vi "Sequence Dialog.vi"(8 "error in (no error)":errorcluster, 10 "Sequence UI":refnum<queue>, 11 "State Cluster In":T3 {"Main Config"."PR Module Configs"."Settings"."PID 2 Parameters"."output range"."output low" format="%.2f"; "Main Config"."PR Module Configs"."Settings"."PID 2 Parameters"."output range"."output high" min=0.0 max=100.0 format="%.2f"; "Main Config"."PR Module Configs"."Settings"."PID 2 Parameters"."PID gains"."derivative time (Td, min)" format="%.3f"; "Main Config"."PR Module Configs"."Settings"."PID 2 Parameters"."PID gains"."integral time (Ti, min)" format="%.3f"; "Main Config"."PR Module Configs"."Settings"."PID 2 Parameters"."PID gains"."proportional gain (Kc)" format="%.3f"; "Main Config"."Steps"."Control" items=["Pump %", "Setpoint"]; "Main Config"."TCU Module Configs"."Settings"."Julabo FP-50 Settings"."Pump Power" min=0 max=8 step=1; "Main Config"."TCU Module Configs"."Settings"."Lauda Settings"."Pump Power" min=0 max=8 step=1; "Main Config"."Pump Module Configs"."Settings"."ASIA Pump C"."channel" min=0 max=1 step=1; "Main Config"."Pump Module Configs"."Settings"."Masterflex"."Pump Number" min=1.0 max=20.0 step=1.0; "Main Config"."Pump Module Configs"."Settings"."Ismatech"."Pump Number" min=1.0 max=20.0 step=1.0; "Main Config"."Feed Module Configs"."Settings"."output range"."output low" min=0.0 max=100.0 format="%.2f"; "Main Config"."Feed Module Configs"."Settings"."output range"."output high" format="%.2f"; "Main Config"."Feed Module Configs"."Settings"."PID 2 Parameters"."PID gains"."derivative time (Td, min)" format="%.3f"; "Main Config"."Feed Module Configs"."Settings"."PID 2 Parameters"."PID gains"."integral time (Ti, min)" format="%.3f"; "Main Config"."Feed Module Configs"."Settings"."PID 2 Parameters"."PID gains"."proportional gain (Kc)" format="%.3f"; "Main Config"."Feed Module Configs"."Settings"."ASIA Pump C"."channel" min=0 max=1 step=1; "Main Config"."Feed Module Configs"."Settings"."Ismatech"."Pump Number" min=1.0 max=20.0 step=1.0; "Main Config"."Feed Module Configs"."Settings"."Masterflex"."Pump Number" min=1.0 max=20.0 step=1.0}) -> (0 "error out":errorcluster, 1 "Start":bool, 2 "cancelled":bool, 3 "State Cluster Out":T3 {"Main Config"."PR Module Configs"."Settings"."PID 2 Parameters"."output range"."output low" format="%.2f"; "Main Config"."PR Module Configs"."Settings"."PID 2 Parameters"."output range"."output high" min=0.0 max=100.0 format="%.2f"; "Main Config"."PR Module Configs"."Settings"."PID 2 Parameters"."PID gains"."derivative time (Td, min)" format="%.3f"; "Main Config"."PR Module Configs"."Settings"."PID 2 Parameters"."PID gains"."integral time (Ti, min)" format="%.3f"; "Main Config"."PR Module Configs"."Settings"."PID 2 Parameters"."PID gains"."proportional gain (Kc)" format="%.3f"; "Main Config"."Steps"."Control" items=["Pump %", "Setpoint"]; "Main Config"."TCU Module Configs"."Settings"."Julabo FP-50 Settings"."Pump Power" min=0 max=8 step=1; "Main Config"."TCU Module Configs"."Settings"."Lauda Settings"."Pump Power" min=0 max=8 step=1; "Main Config"."Pump Module Configs"."Settings"."ASIA Pump C"."channel" min=0 max=1 step=1; "Main Config"."Pump Module Configs"."Settings"."Masterflex"."Pump Number" min=1.0 max=20.0 step=1.0; "Main Config"."Pump Module Configs"."Settings"."Ismatech"."Pump Number" min=1.0 max=20.0 step=1.0; "Main Config"."Feed Module Configs"."Settings"."output range"."output low" min=0.0 max=100.0 format="%.2f"; "Main Config"."Feed Module Configs"."Settings"."output range"."output high" format="%.2f"; "Main Config"."Feed Module Configs"."Settings"."PID 2 Parameters"."PID gains"."derivative time (Td, min)" format="%.3f"; "Main Config"."Feed Module Configs"."Settings"."PID 2 Parameters"."PID gains"."integral time (Ti, min)" format="%.3f"; "Main Config"."Feed Module Configs"."Settings"."PID 2 Parameters"."PID gains"."proportional gain (Kc)" format="%.3f"; "Main Config"."Feed Module Configs"."Settings"."ASIA Pump C"."channel" min=0 max=1 step=1; "Main Config"."Feed Module Configs"."Settings"."Ismatech"."Pump Number" min=1.0 max=20.0 step=1.0; "Main Config"."Feed Module Configs"."Settings"."Masterflex"."Pump Number" min=1.0 max=20.0 step=1.0}, 4 "Pause":bool, 5 "Abort":bool)   [LabVIEW 2018, in "Sequencing Library.lvlib"]
uses:
  Sequencing Library.lvlib
  Squence Control.ctl
  controls/Step Cluster.ctl
  Drag and Drop/State Cluster.ctl
  support/Message Queue/Message Cluster.ctl
  Drag and Drop/Thumbnail Cluster.ctl
  Drag and Drop/Object Cluster.ctl
  <vilib>/Utility/miscctls.llb/LVRectTypeDef.ctl
  Drag and Drop/Object Type Enum.ctl
  <vilib>/Utility/miscctls.llb/LVPositionTypeDef.ctl
  Config Module/Controls/Main Config Cluster.ctl
  OPC/OPC Module Config.ctl
  Scale Module Folder/Measure Instrument/State Enum.ctl
  <vilib>/Utility/miscctls.llb/LVPoint32TypeDef.ctl
  OPC/OPC Settings.ctl
  OPC/Variable Data Cluster.ctl
  <vilib>/OPCUA/controls/NodeId.ctl
  <vilib>/OPCUA/controls/OPC UA StatusCode.ctl
  <vilib>/OPCUA/controls/Subscription ID.ctl
  <vilib>/OPCUA/controls/OPC UA Client Refnum.ctl
  <vilib>/OPCUA/controls/Subscription Data Change.ctl
  <vilib>/OPCUA/controls/Data Type.ctl
  Feed Module/Controls/Feed Module Config Cluster.ctl
  Feed Module/Controls/Feed Module Settings Cluster.ctl
  Ismatec ISM 831C/Controls/Ismatech Settings Cluster.ctl
  Masterflex 7550-30/Controls/Settings Cluster.ctl
  Mettler Toledo/Controls/Settings Cluster.ctl
  Bronkhorst M13 Flow Meter/Settings Cluster.ctl
  Measure Instrument/PID 2 Parameters Cluster.ctl
  Measure Instrument/PID Input Enum.ctl
  Measure Instrument/PID 2 Output Enum.ctl
  Tacmina QI/Tacmina QI DAQ Setting.ctl
  KNF Pump/Settings Cluster plus SIMDOS.ctl
  ASIA Pump/Pump Settings.ctl
  VICI M50 Party Mode/Settings Cluster.ctl
  FLOM Pump/Settings Cluster.ctl
  SSI PR Class/SSI PR or LD Settings Cluster.ctl
  Masterflex 75211/Masterflex 75211 DAQ Setting.ctl
  SSI PR Class/SSI P40 Settings Cluster.ctl
  TT Module/Controls/TT Module Config Cluster.ctl
  Tag VIs/Numeric Alarm Settings Cluster.ctl
  Acquisition/Hardware Configuration.ctl
  Acquisition/Task Cluster.ctl
  PT Module/Controls/PT Module Config Cluster.ctl
  Scale Module Folder/Feed Module/Controls/Scale Module Config Cluster.ctl
  Scale Module Folder/Feed Module/Controls/Scale Module Settings Cluster.ctl
  Pump Module Folder/Pump Module Config Cluster.ctl
  Pump Module Folder/Pump Module Settings Cluster.ctl
  LabJack Module/Controls/U3 Module Config Cluster.ctl
  Decoration Module/Decoration Module Config Cluster.ctl
  Flow Module Folder/Feed Module/Controls/Flow Module Config Cluster.ctl
  Flow Module Folder/Feed Module/Controls/Flow Module Settings Cluster.ctl
  TCU Module/TCU Module Folder/TCU Module Config Cluster.ctl
  TCU Module/TCU Module Folder/TCU Module Settings Cluster.ctl
  TCU Module/TCU Module Folder/Measure Instrument/Output Devices.ctl
  Huber TCU/Huber Settings.ctl
  Lauda Integral XT-150 TCU/Lauda Settings.ctl
  Julabo Type 1 TCU/Julabo Type 1 TCU Folder/Julabo FP-50 Settings.ctl
  Huber Unistat 410 TCU/Huber Unistat 410 Settings.ctl
  D-O Module Folder/Not Sure Where this is Used.ctl
  D-O Module Folder/D-O Module Config Cluster.ctl
  D-O Module Folder/Valve Clusters.ctl
  D-O Module Folder/D-O Module Settings Cluster.ctl
  D-O Module Folder/D-O Device Settings Cluster.ctl
  VICI Electronic Actuator/VICI Electronic Actuator Settings.ctl
  Pressure Regulator Control Module/Pressure Regulator/Controls/4-20mA Module Config Cluster.ctl
  Pressure Regulator Control Module/Pressure Regulator/Controls/4-20mA Module Settings Cluster.ctl
  Pressure Transmitter/Pressure Transmitter Device Settings.ctl
  Pressure Reg Module/Pressure Regulator Device Settings.ctl
  support/Message Queue/Enqueue Message (Single).vi
  support/Message Queue/Message Queue.lvlib
  Drag and Drop/Drag and Drop.lvlib
  Config Module/Config Module.lvlib
  TT Module/TT Module.lvlib
  Feed Module/Feed Module.lvlib
  Ismatec ISM 831C/Ismatec ISM 831C.lvlib
  Masterflex 7550-30/Masterflex 7550-30.lvlib
  Mettler Toledo/Mettler Toledo.lvlib
  Bronkhorst M13 Flow Meter/Bronkhorst M13 Flow Meter.lvlib
  Tacmina QI/Tacmina QI.lvlib
  KNF Pump/KNF SIMDOS.lvlib
  ASIA Pump.lvlib
  DAQ/DAQ.lvlib
  PT Module/PT Module.lvlib
  Scale Module Folder/Scale Module.lvlib
  Pump Module Folder/Pump Module.lvlib
  LabJack Module/U3 Module.lvlib
  Flow Module Folder/Flow Module.lvlib
  TCU Module/TCU Module Folder/TCU Module.lvlib
  Huber TCU/Huber Ministat 230 TCU.lvlib
  Lauda Integral XT-150 TCU/Lauda TCU.lvlib
  Julabo Type 1 TCU/Julabo Type 1 TCU Folder/Julabo Type FP-50 TCU.lvlib
  VICI M50 Party Mode/VICI M6 M50 Party Mode.lvlib
  D-O Module Folder/D-O Module.lvlib
  Pressure Transmitter/Pressure Transmitter Library.lvlib
  Pressure Regulator Control Module/Pressure Regulator/4-20mA Module.lvlib
  Pressure Reg Module/Pressure Regulator Library.lvlib
  FLOM Pump/FLOM Pump.lvlib
  SSI PR Class/SSI PR or LD Pump.lvlib
  Huber Unistat 410 TCU/Huber Unistat 410 TCU.lvlib
  OPC/OPC UA.lvlib
  Scale Module Folder/Measure Instrument/Scale Module Engine.lvlib
  D-O Module Folder/DIO Valve/VICI Electronic Actuator.lvlib
  Masterflex 75211/Masterflex 75211.lvlib
  SSI PR Class/SSI P40 Pump.lvlib
panel:
  out "Main Config.Steps":T1 {"Control" items=["Pump %", "Setpoint"]}
  out "Strings []":string[](array[string])
  in  "Abort  Button":bool
  in  "Pause Button":bool
  in  "Save Button":bool
  in  "Step Array":T65[](array[typedef]) {"Value" min=0.0 max=100.0; "Control" items=["Pump Module Setpoint", "Feed Module Setpoint", "Digital On/Off", "Wait Until Output <=", "Wait Until Output >=", "TCU Pump Setpoint", "TCU Temperature Setpoint", "Wait until TCU Temp <=", "Wait until TCU Temp >=", "Default"]; "Module" items=["Default", "Start Loop", "End Loop", "PM1"]}
  out "Steps out":T2[](array[typedef]) {"Control" items=["Setpoint", "Pump %"]}
  in  "Cancel Button":bool
  in  "Start Button":bool
  # "Module"
  # "Control"
  # "Value"
  # "Wait (sec)"
  # "Running"
  # "Instrument Settings"
  # "Instrument Settings"
  # "Output Instruments"
  # "Flow Meter Settings"
  # "Output Instruments"
  # "Scale Settings"
  # "Output Instruments"
  # "Input Instruments"
  # "Instrument Settings"
  # "Instrument Settings"
  # "Output Instruments"
  # "Flow Meter Settings"
  # "Output Instruments"
  # "Scale Settings"
  # "Output Instruments"
  # "Input Instruments"
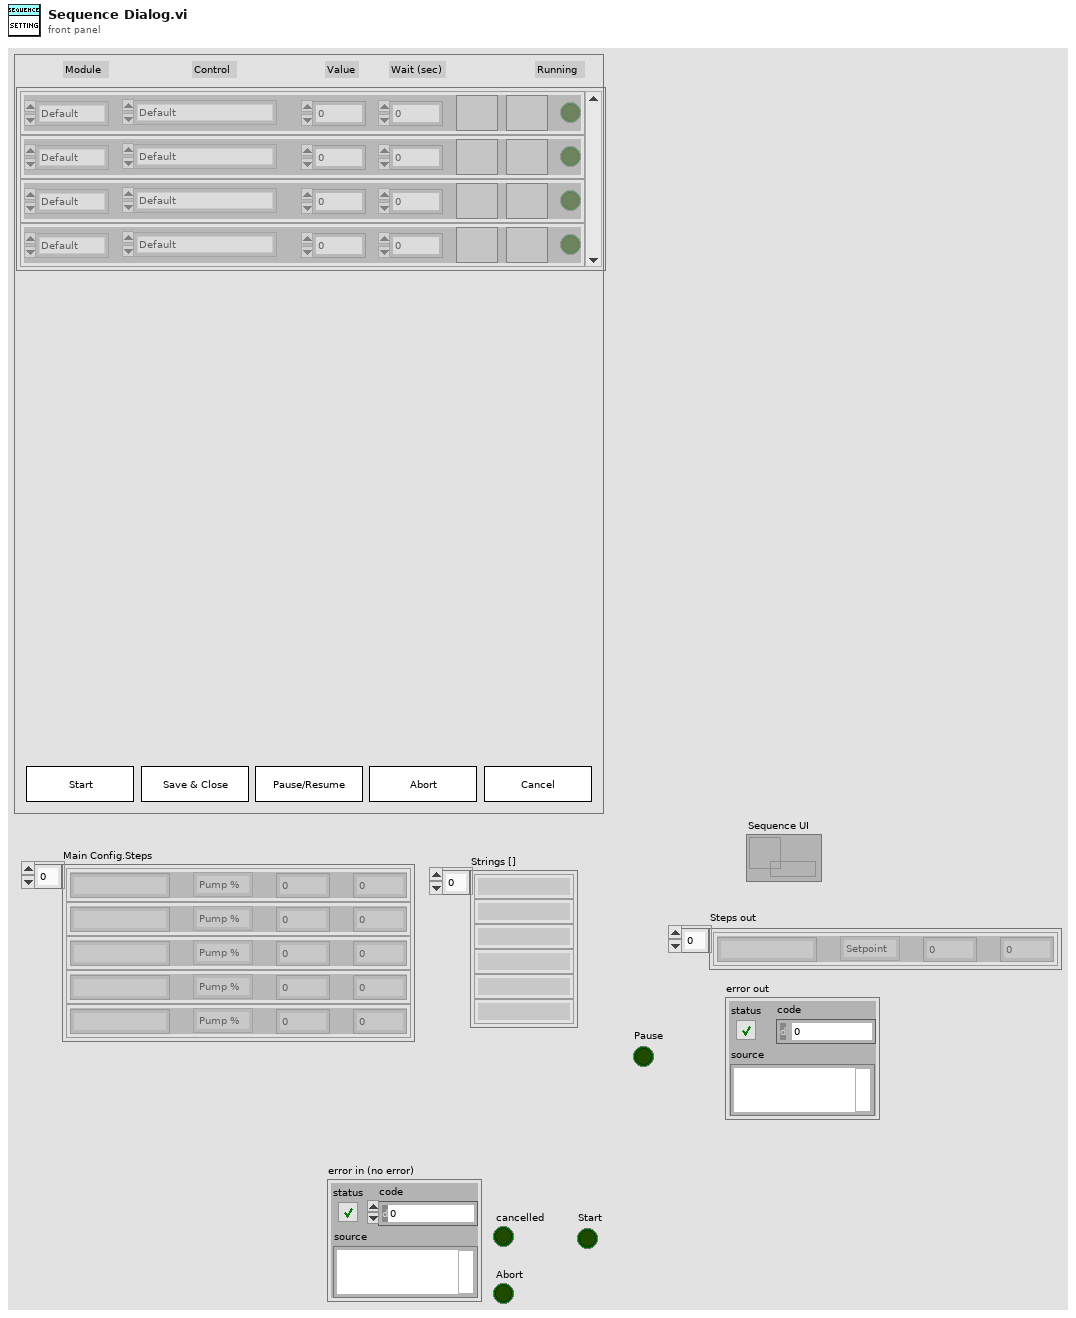
[diagram p1: front panel]
types:
  T1 = typedef "Not Sure Where this is Used.ctl" = T2[]
  T2 = typedef "Sequencing Library.lvlib/Squence Control.ctl" = cluster{"Module":string, "Control":u16, "Value":dbl, "Wait (sec)":dbl}
  T3 = typedef "Drag and Drop.lvlib/State Cluster.ctl" = cluster{"VI refs":refnum<vi>[], "Queues":refnum<queue>[], "[Thumbnails]":T4[], "Drag Object Idx":i32, "[Objects]":T5[], "Active Object":i32, "Drop Offset":T8, "Process Name":string, "Main Config":T9, "Campaign Filepath":path, "Config Changed?":bool}
  T4 = typedef "Thumbnail Cluster.ctl" = cluster{"Path":path, "Rectangle":cluster{"left":i16, "top":i16, "right":i16, "bottom":i16}}
  T5 = typedef "Object Cluster.ctl" = cluster{"BMP Path":path, "Anchor Position":cluster{"X":i32, "Y":i32}, "Hot Spot":T6, "Type":T7, "Parameters":variant}
  T6 = typedef "LVRectTypeDef.ctl" = cluster{"Left":i16, "Top":i16, "Right":i16, "Bottom":i16}
  T7 = typedef "Object Type Enum.ctl" = enum16{"Icon", "Line", "Text", "Feed Module"}
  T8 = typedef "LVPositionTypeDef.ctl" = cluster{"Left":i32, "Top":i32}
  T9 = typedef "Config Module.lvlib/Main Config Cluster.ctl" = cluster{"Notebook":string, "Page":string, "OPC Module Configs":T10[], "Feed Module Configs":T19[], "Log File Path":path, "TT Module Configs":T36[], "DAQ Config":T38, "PT Module Configs":T40[], "Scale Module Configs":T41[], "Pump Module Configs":T43[], "U3 Module Configs":T45[], "Decoration Module Configs":T46[], "Flow Module Configs":T47[], "TCU Module Configs":T49[], "Steps":T1, "Abort":bool, "DO Module Configs":T56[], "PR Module Configs":T61[], "Cycle Period":dbl}
  T10 = typedef "OPC UA.lvlib/OPC Module Config.ctl" = cluster{"State":T11, "GUID":string, "Drop Coords":T12, "Configuration":T13, "First Iteration":bool, "Data":cluster{"Object Name":string, "Variable Array":T14[]}[], "Process Name":string, "Load Count":i32, "Log Started":bool, "subscription ID out":T17, "OPC UA client refnum out":T18, "Event Registration Refnum":refnum<event-registration>, "Start Time":timestamp, "Current Time":timestamp}
  T11 = typedef "Scale Module.lvlib/Scale Module Engine.lvlib/State Enum.ctl" = enum16{"Measuring", "Idle"}
  T12 = typedef "LVPoint32TypeDef.ctl" = cluster{"Horizontal":i32, "Vertical":i32}
  T13 = typedef "OPC UA.lvlib/OPC Settings.ctl" = cluster{"Cycle Period":dbl, "server endpoint URL":string, "security policy":cluster{"message mode":enum16{"None", "Sign", "Sign and Encrypt"}, "security":enum16{"Basic256", "Basic128Rsa15"}}, "Trust Any Server":bool}
  T14 = typedef "OPC UA.lvlib/Variable Data Cluster.ctl" = cluster{"node ID":T15, "browse name":string, "status":T16, "timestamp":timestamp, "value ":variant}
  T15 = typedef "NodeId.ctl" = string
  T16 = typedef "OPC UA StatusCode.ctl" = u32
  T17 = typedef "Subscription ID.ctl" = u32
  T18 = typedef "OPC UA Client Refnum.ctl" = refnum<k21>
  T19 = typedef "Feed Module.lvlib/Feed Module Config Cluster.ctl" = cluster{"GUID":string, "Drop Coords":T12, "Process Name":string, "Queue Name":string, "Settings":T20, "Settings Load Count":i32, "OP Load Count":i32}
  T20 = typedef "Feed Module.lvlib/Feed Module Settings Cluster.ctl" = cluster{"Cycle Period":dbl, "Ismatech":T21, "Masterflex":T22, "Mettler":T23, "Bronkhorst M13 Flow Meter":T24, "PID 2 Parameters":T25, "Manual Entry":dbl, "Auto?":bool, "output range":cluster{"output high":dbl, "output low":dbl}, "Bronkhorst M14":T23, "Tacmina Settings":T28, "KNF SIMDOS Settings":T29, "ASIA Pump C":T30, "VICI Settings":T31, "FLOM Settings":T32, "SSI PR/LD Settings":T33, "Masterflex 75211 Settings":T34, "SSI P40 Settings":T35}
  T21 = typedef "Ismatec ISM 831C.lvlib/Ismatech Settings Cluster.ctl" = cluster{"VISA resource name":refnum<visa-resource-name>, "Simulated?":bool, "Pump Number":dbl, "Reverse?":bool}
  T22 = typedef "Masterflex 7550-30.lvlib/Settings Cluster.ctl" = cluster{"VISA resource name":refnum<visa-resource-name>, "Simulated?":bool, "Pump Number":dbl, "Reverse?":bool}
  T23 = typedef "Mettler Toledo.lvlib/Settings Cluster.ctl" = cluster{"VISA resource name":refnum<visa-resource-name>, "Simulated?":bool}
  T24 = typedef "Bronkhorst M13 Flow Meter.lvlib/Settings Cluster.ctl" = cluster{"VISA resource name":refnum<visa-resource-name>, "Simulated?":bool}
  T25 = typedef "PID 2 Parameters Cluster.ctl" = cluster{"Input Device":T26, "Output Device":T27, "Setpoint":dbl, "PID gains":cluster{"proportional gain (Kc)":dbl, "integral time (Ti, min)":dbl, "derivative time (Td, min)":dbl}}
  T26 = typedef "PID Input Enum.ctl" = enum16{"Default", "Bronkhorst M13", "Bronkhorst M14", "Scale Rate of Change"}
  T27 = typedef "PID 2 Output Enum.ctl" = enum16{"Default", "Ismatec ISM 831C", "Masterflex 7550-30", "VICI", "Tacmina QI", "KNF SIMDOS", "ASIA Type C", "FLOM UI-22-11", "SSI PR/LD", "SSI P40", "Masterflex 75211-70"}
  T28 = typedef "Tacmina QI.lvlib/Tacmina QI DAQ Setting.ctl" = cluster{"Analog DAQ Task":refnum<k21>, "Digital DAQ Task":refnum<k21>}
  T29 = typedef "KNF SIMDOS.lvlib/Settings Cluster plus SIMDOS.ctl" = cluster{"VISA resource name":refnum<visa-resource-name>, "Simulated?":bool}
  T30 = typedef "ASIA Pump.lvlib/Pump Settings.ctl" = cluster{"ASIA Pump #":i32, "channel":i32, "Simulated":bool}
  T31 = typedef "VICI M6 M50 Party Mode.lvlib/Settings Cluster.ctl" = cluster{"VISA resource name":refnum<visa-resource-name>, "Simulated?":bool, "Pump Letter":string, "Reverse?":bool}
  T32 = typedef "FLOM Pump.lvlib/Settings Cluster.ctl" = cluster{"VISA resource name":refnum<visa-resource-name>, "Simulated?":bool, "Pump Number":dbl}
  T33 = typedef "SSI PR or LD Pump.lvlib/SSI PR or LD Settings Cluster.ctl" = cluster{"VISA resource name":refnum<visa-resource-name>, "Simulated?":bool}
  T34 = typedef "Masterflex 75211.lvlib/Masterflex 75211 DAQ Setting.ctl" = cluster{"Analog DAQ Task":refnum<k21>, "Digital DAQ Task":refnum<k21>}
  T35 = typedef "SSI P40 Pump.lvlib/SSI P40 Settings Cluster.ctl" = cluster{"VISA resource name":refnum<visa-resource-name>, "Simulated?":bool}
  T36 = typedef "TT Module.lvlib/TT Module Config Cluster.ctl" = cluster{"GUID":string, "Drop Coords":T12, "Input Channel Tag Name ":string, "Process Name":string, "Queue Name":string, "Input Channel Numeric Alarm Settings":T37[]}
  T37 = typedef "Numeric Alarm Settings Cluster.ctl" = cluster{"enable? (F)":bool, "name":string, "alarm type":enum16{"HI_HI", "HI", "LO", "LO_LO"}, "level/change":dbl, "deadband/time":dbl, "alarm delay":dbl, "priority":u32, "ack type":enum16{"Auto", "User", "None", "Each Occurrence"}, "area":string, "description":string, "log? (T)":bool}
  T38 = typedef "DAQ.lvlib/Hardware Configuration.ctl" = cluster{"Tasks":T39[]}
  T39 = typedef "Task Cluster.ctl" = cluster{"DAQmx Task":refnum<k21>, "Read-Write Radio":enum32{"Read", "Write"}}
  T40 = typedef "PT Module.lvlib/PT Module Config Cluster.ctl" = cluster{"GUID":string, "Drop Coords":T12, "Input Channel Tag Name ":string, "Process Name":string, "Queue Name":string, "Input Channel Numeric Alarm Settings":T37[]}
  T41 = typedef "Scale Module.lvlib/Scale Module Config Cluster.ctl" = cluster{"GUID":string, "Drop Coords":T12, "Process Name":string, "Queue Name":string, "Settings":T42, "Load Count":i32}
  T42 = typedef "Scale Module.lvlib/Scale Module Settings Cluster.ctl" = cluster{"Cycle Period":dbl, "Mettler":T23, "Scale Type":string}
  T43 = typedef "Pump Module.lvlib/Pump Module Config Cluster.ctl" = cluster{"GUID":string, "Drop Coords":T12, "Process Name":string, "Queue Name":string, "Settings":T44, "Load Count":i32}
  T44 = typedef "Pump Module.lvlib/Pump Module Settings Cluster.ctl" = cluster{"Cycle Period":dbl, "Manual Entry":dbl, "Output Device":T27, "Ismatech":T21, "Masterflex":T22, "VICI Settings":T31, "Tacmina Settings":T28, "KNF SIMDOS Settings":T29, "ASIA Pump C":T30, "FLOM Settings":T32, "SSI PR/LD Settings":T33, "SSI P40 Settings":T33, "Masterflex 75211 Settings":T34, "Pump Calibration File":path, "Calibration Slope":dbl, "Calibration Y Intercept":dbl, "Pump Cal Enum":u16}
  T45 = typedef "U3 Module.lvlib/U3 Module Config Cluster.ctl" = cluster{"GUID":string, "Drop Coords":T12, "AI Channel Number":enum16{"Default", "AI0", "AI1", "AI2", "AI3", "AI4", "AI5", "AI6", "AI7"}, "Process Name":string, "Queue Name":string, "Input Channel Numeric Alarm Settings":T37[]}
  T46 = typedef "Decoration Module Config Cluster.ctl" = cluster{"GUID":string, "Drop Coords":T12, "Decoration Filepath":path}
  T47 = typedef "Flow Module.lvlib/Flow Module Config Cluster.ctl" = cluster{"GUID":string, "Drop Coords":T12, "Process Name":string, "Queue Name":string, "Settings":T48, "Load Count":i32}
  T48 = typedef "Flow Module.lvlib/Flow Module Settings Cluster.ctl" = cluster{"Cycle Period":dbl, "Bronkhorst M13":T23, "Flow Meter Type":string, "Bronkhorst M14":T23}
  T49 = typedef "TCU Module.lvlib/TCU Module Config Cluster.ctl" = cluster{"GUID":string, "Drop Coords":T12, "Process Name":string, "Queue Name":string, "Settings":T50, "Load Count":i32, "Power Level Changed":bool}
  T50 = typedef "TCU Module.lvlib/TCU Module Settings Cluster.ctl" = cluster{"Cycle Period":dbl, "Setpoint Entry":dbl, "Output Device":T51, "Huber Ministat 230 Settings":T52, "Lauda Settings":T53, "Julabo FP-50 Settings":T54, "Internal Control?":bool, "Huber Unistat 410 Settings":T55}
  T51 = typedef "Output Devices.ctl" = enum16{"Default", "Huber Ministat 230", "Huber Unistat 410", "Lauda XT-150", "Julabo FP-50"}
  T52 = typedef "Huber Ministat 230 TCU.lvlib/Huber Settings.ctl" = cluster{"VISA resource name":refnum<visa-resource-name>, "Simulated?":bool}
  T53 = typedef "Lauda TCU.lvlib/Lauda Settings.ctl" = cluster{"VISA resource name":refnum<visa-resource-name>, "Simulated?":bool, "Pump Power":i32}
  T54 = typedef "Julabo Type FP-50 TCU.lvlib/Julabo FP-50 Settings.ctl" = cluster{"VISA resource name":refnum<visa-resource-name>, "Simulated?":bool, "Pump Power":i32}
  T55 = typedef "Huber Unistat 410 TCU.lvlib/Huber Unistat 410 Settings.ctl" = cluster{"VISA resource name":refnum<visa-resource-name>, "Simulated?":bool}
  T56 = typedef "D-O Module.lvlib/D-O Module Config Cluster.ctl" = cluster{"GUID":string, "Drop Coords":T12, "Process Name":string, "Queue Name":string, "Settings":T57, "Load Count":i32}
  T57 = typedef "D-O Module.lvlib/Valve Clusters.ctl" = cluster{"Valve Settings":T58, "Valve Type":enum16{"Default", "Digital Output Valve", "VICI Electronic Actuator"}, "Time On (Sec)":dbl, "Time Off (Sec)":dbl, "Run?":bool}
  T58 = typedef "D-O Module.lvlib/D-O Module Settings Cluster.ctl" = cluster{"D-O Settings":T59, "VICI Electronic Actuator":T60}
  T59 = typedef "D-O Module.lvlib/D-O Device Settings Cluster.ctl" = cluster{"DAQmx Task Name":refnum<k21>, "Output Channel":u16, "Output Channel Names":string[]}
  T60 = typedef "VICI Electronic Actuator.lvlib/VICI Electronic Actuator Settings.ctl" = cluster{"VISA resource name":refnum<visa-resource-name>, "Mode":enum16{"Two Positions With Stops", "Two Positions Without Stops", "Mutiposition"}, "Simulated":bool}
  T61 = typedef "4-20mA Module.lvlib/4-20mA Module Config Cluster.ctl" = cluster{"GUID":string, "Drop Coords":T12, "Process Name":string, "Queue Name":string, "Settings":T62, "Settings Load Count":i32}
  T62 = typedef "4-20mA Module.lvlib/4-20mA Module Settings Cluster.ctl" = cluster{"Cycle Period":dbl, "PID 2 Parameters":cluster{"Input Device":enum16{"Default", "4-20mA"}, "Output Device":enum16{"Default", "Equilibar Pressure Reg", "Flow Regulator"}, "Setpoint":dbl, "PID gains":cluster{"proportional gain (Kc)":dbl, "integral time (Ti, min)":dbl, "derivative time (Td, min)":dbl}, "output range":cluster{"output low":dbl, "output high":dbl}}, "Manual Entry":dbl, "Auto?":bool, "4-20mA Input Settings":T63, "4-20mA Out Settings":T64, "Input Channel Tag Name ":string}
  T63 = typedef "Pressure Transmitter Library.lvlib/Pressure Transmitter Device Settings.ctl" = cluster{"Input Channel ":u16}
  T64 = typedef "Pressure Regulator Library.lvlib/Pressure Regulator Device Settings.ctl" = cluster{"Output DAQ Task":refnum<k21>}
  T65 = typedef "Sequencing Library.lvlib/Step Cluster.ctl" = cluster{"Add Button":bool, "Remove Button":bool, "Module":u16, "Control":u16, "Value":dbl, "Wait (sec)":dbl, "Step Running":bool}
  T66 = cluster{"Add Button":bool, "Remove Button":bool, "Module":u16, "Control":u16, "Value":dbl, "Wait (sec)":dbl, "Step Running":bool}
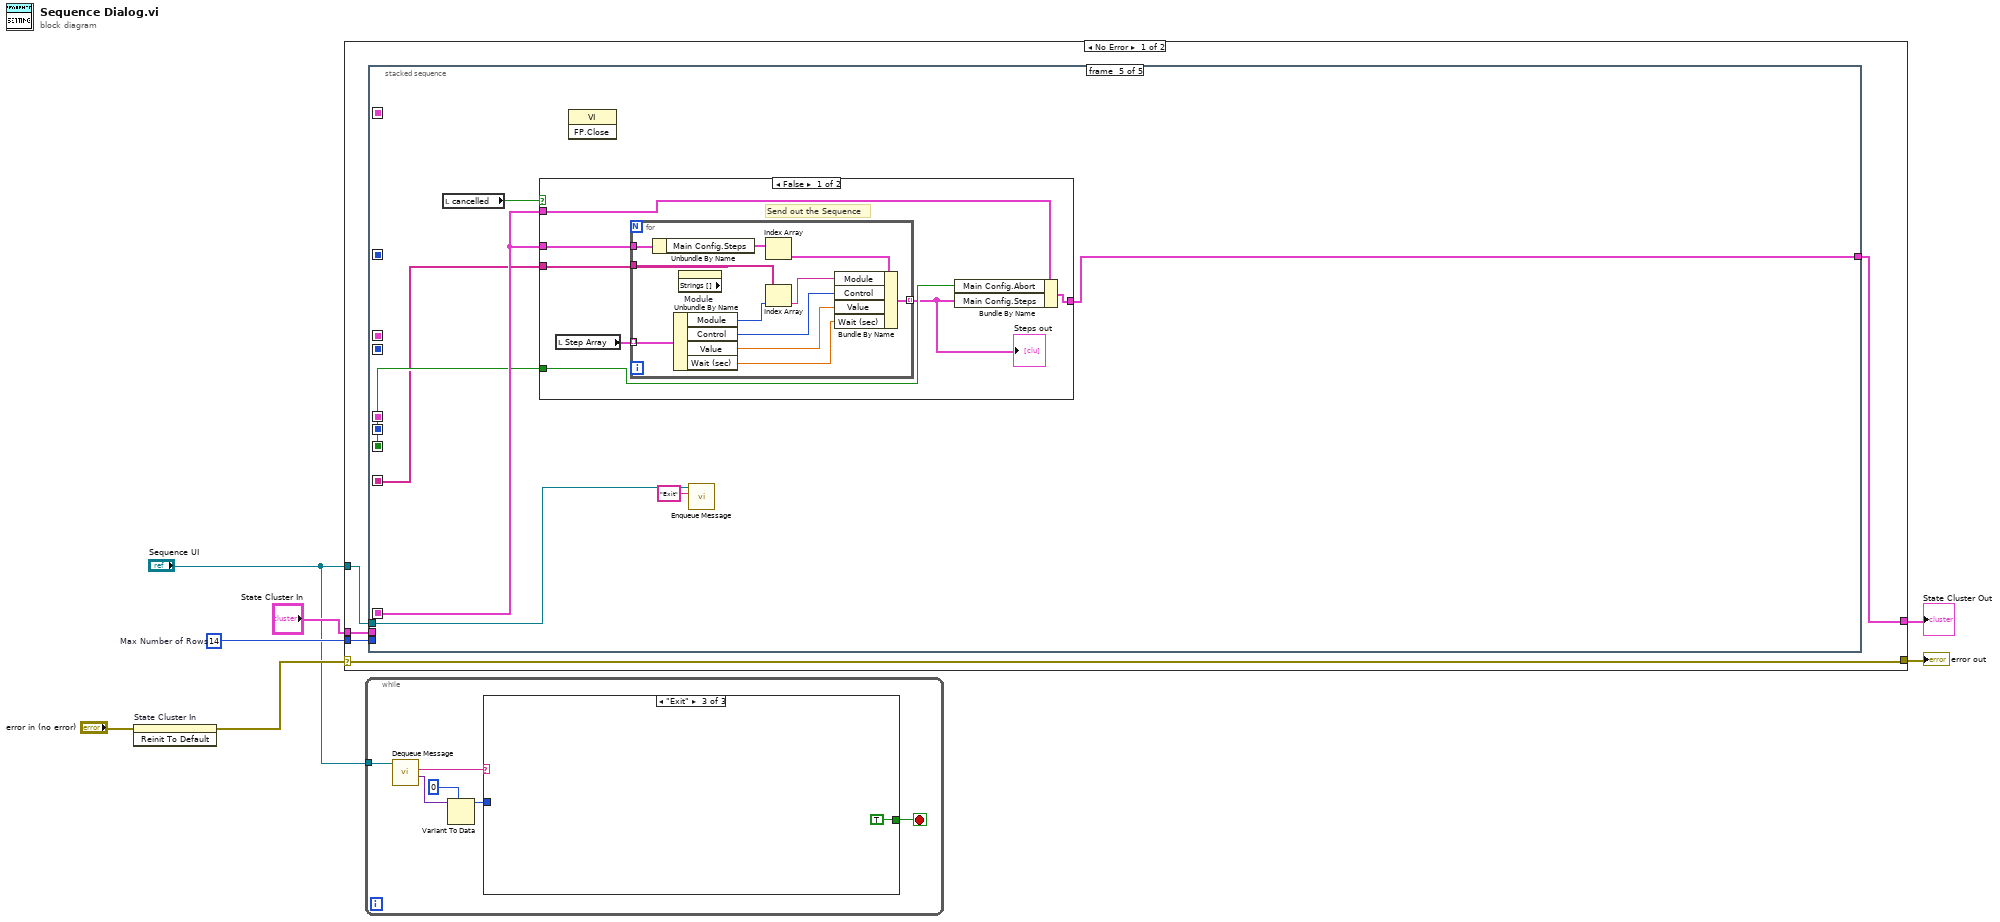
[diagram p0: block diagram]
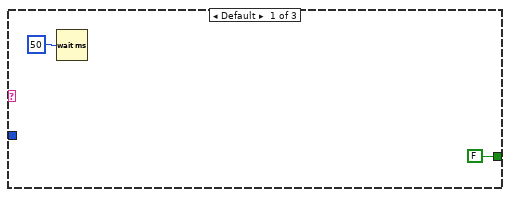
[diagram p2: hidden frame]
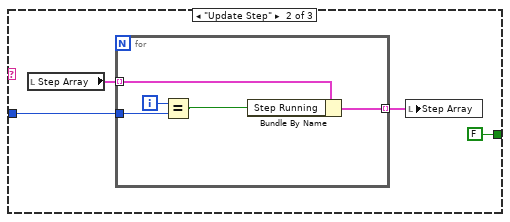
[diagram p3: hidden frame]
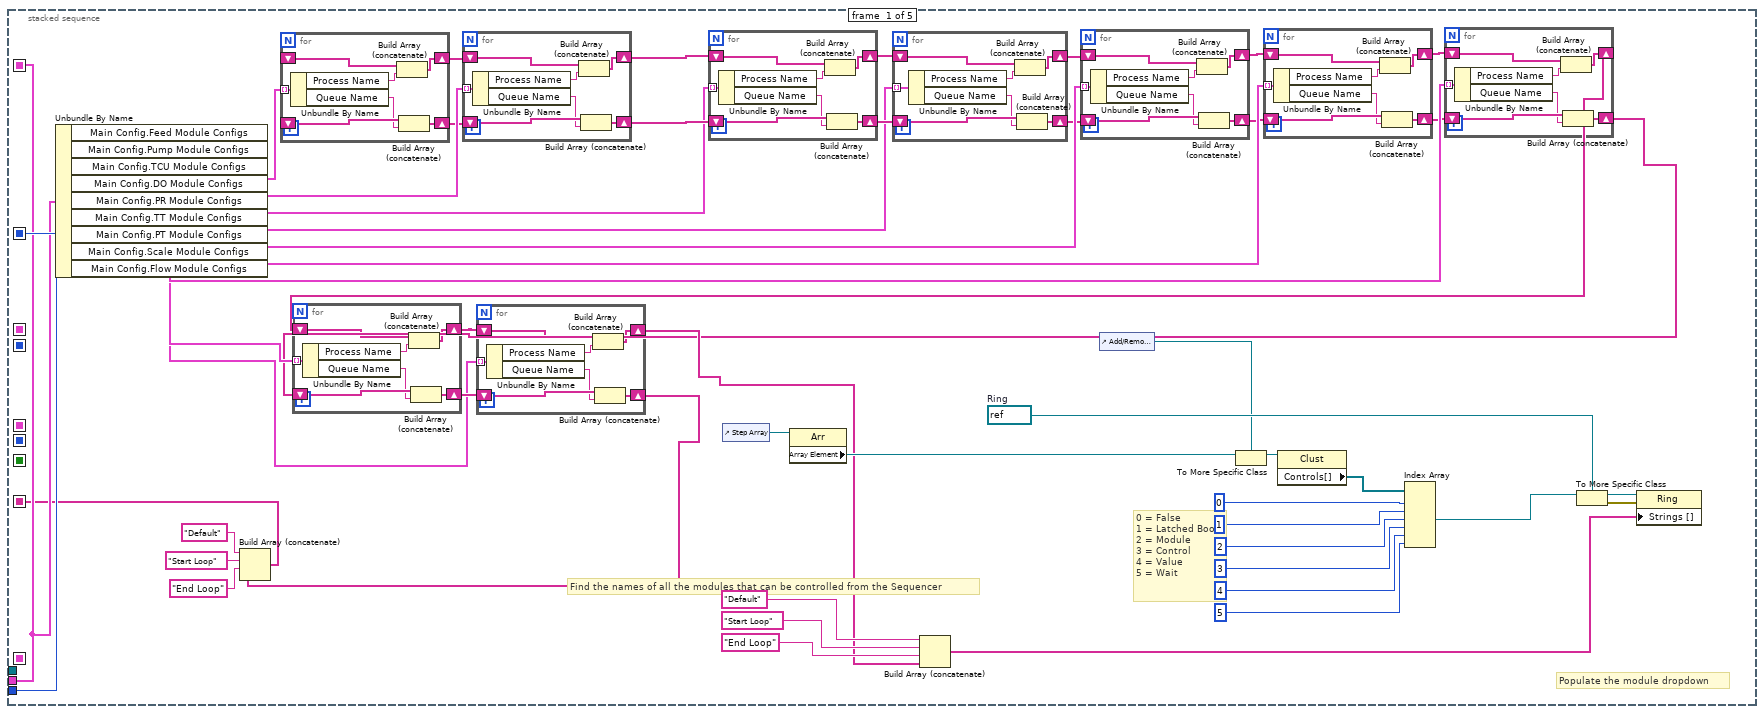
[diagram p4: hidden frame]
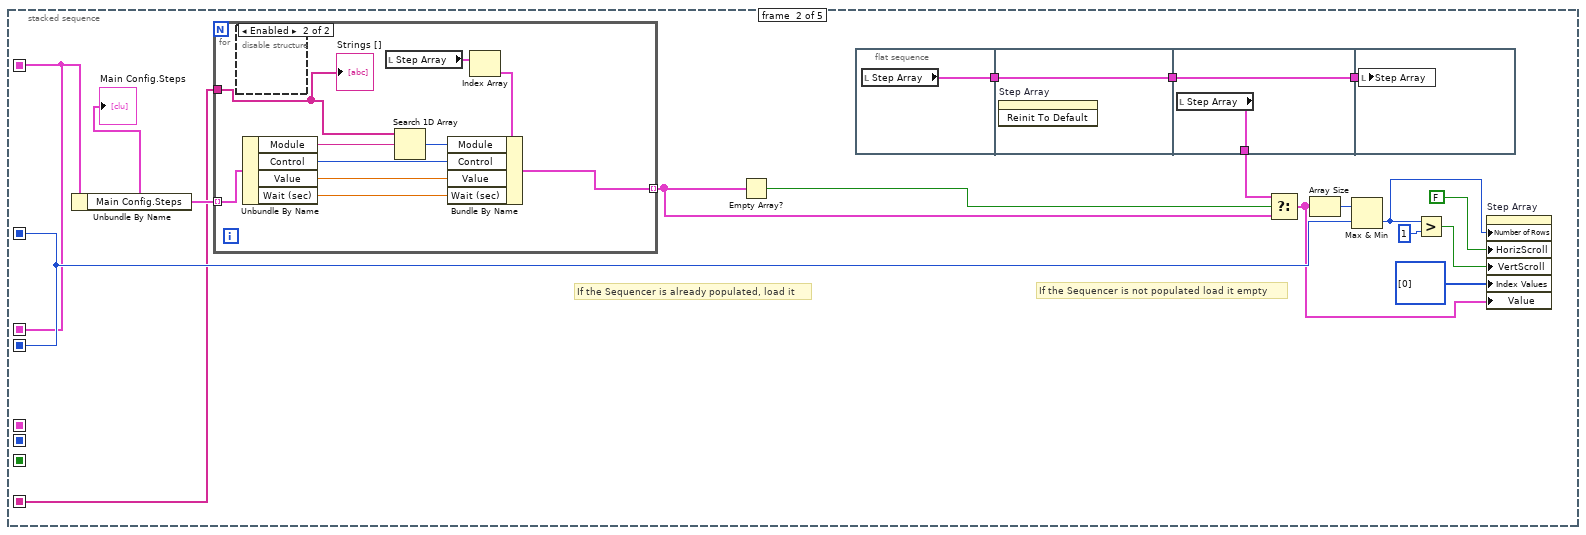
[diagram p5: hidden frame]
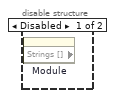
[diagram p6: hidden frame]
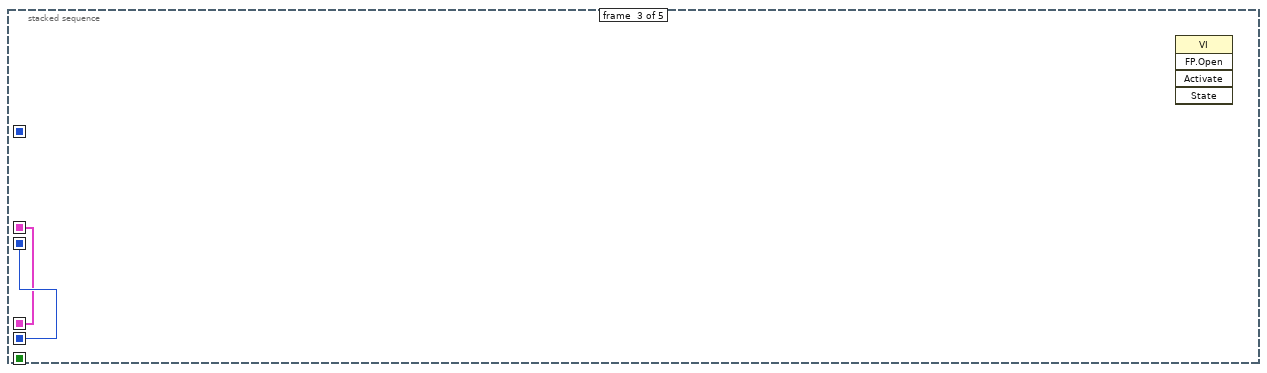
[diagram p7: hidden frame]
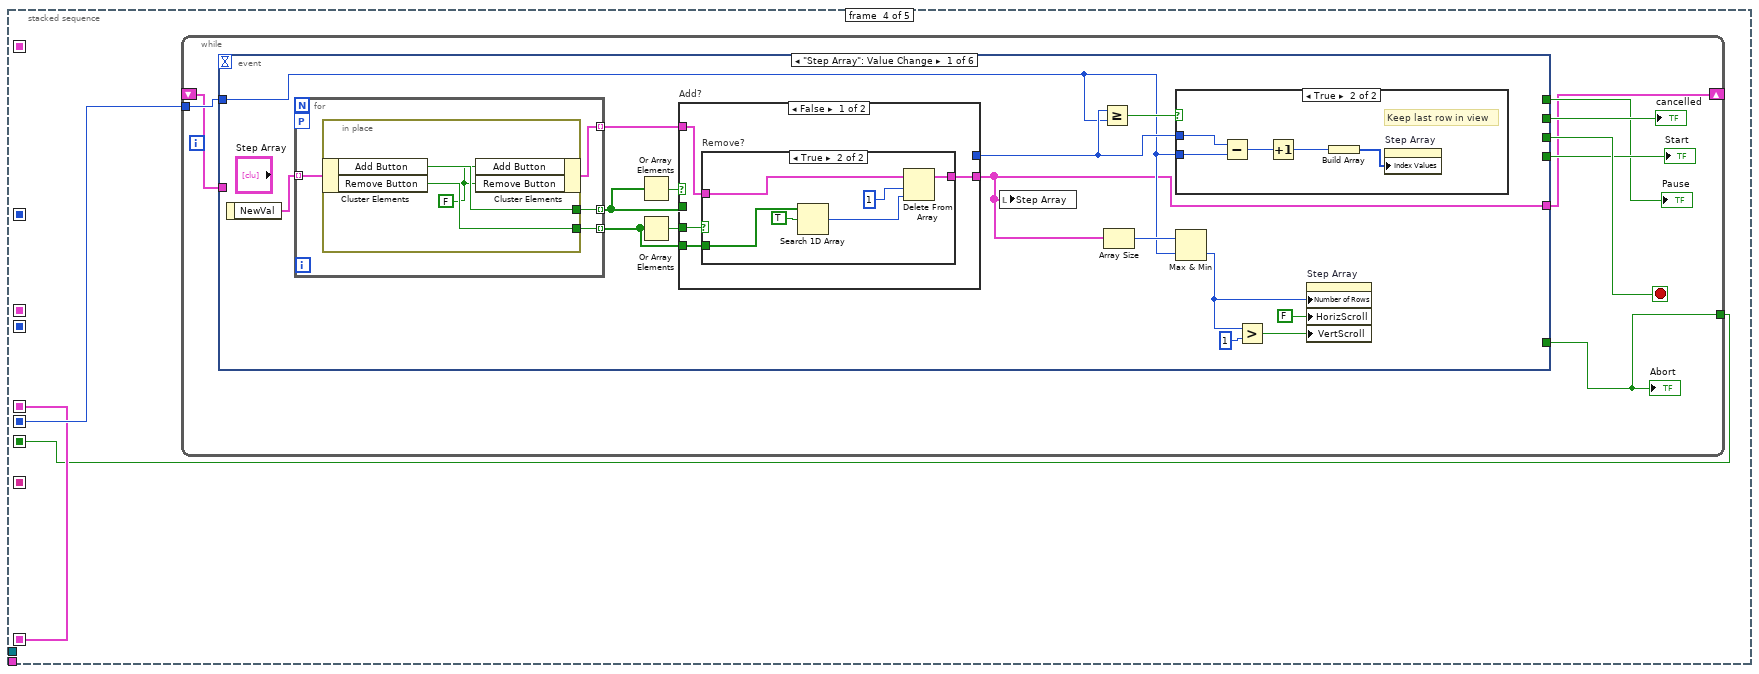
[diagram p8: hidden frame]
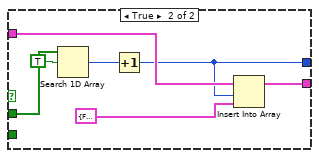
[diagram p11: hidden frame]
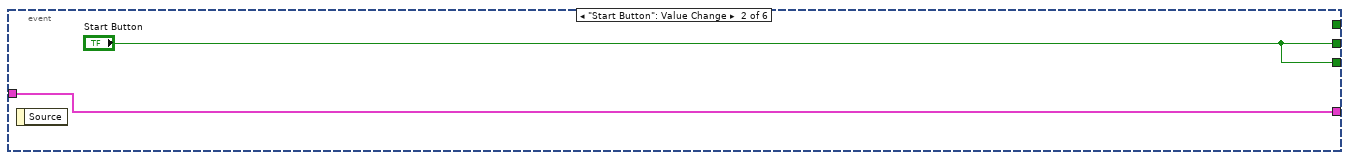
[diagram p12: hidden frame]
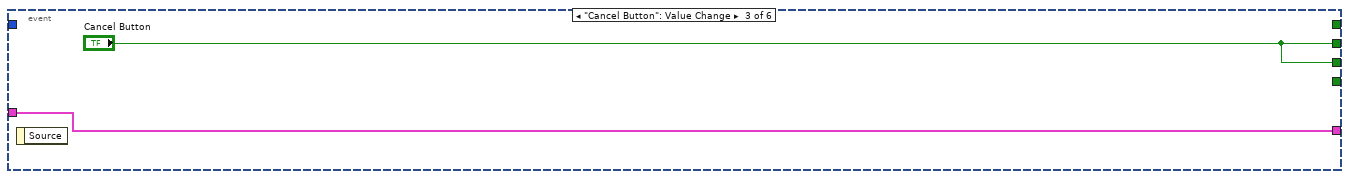
[diagram p13: hidden frame]
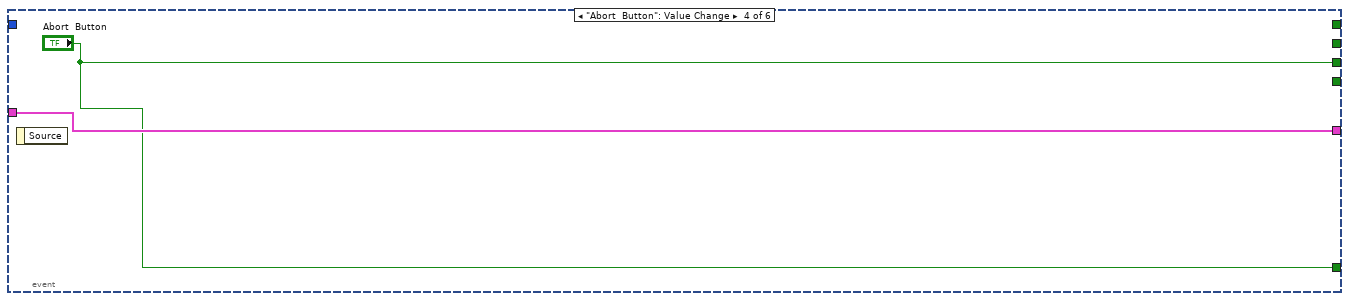
[diagram p14: hidden frame]
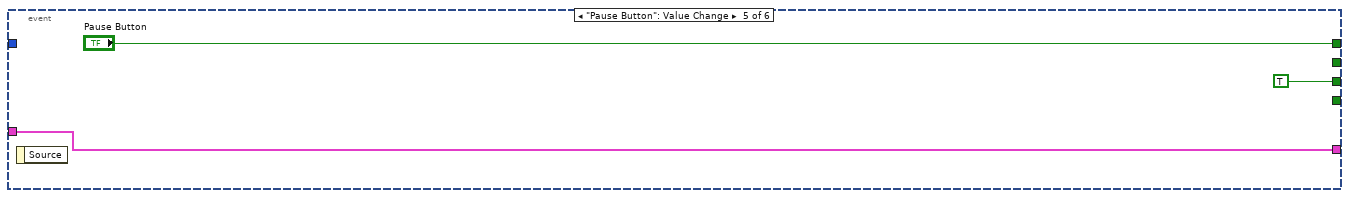
[diagram p15: hidden frame]
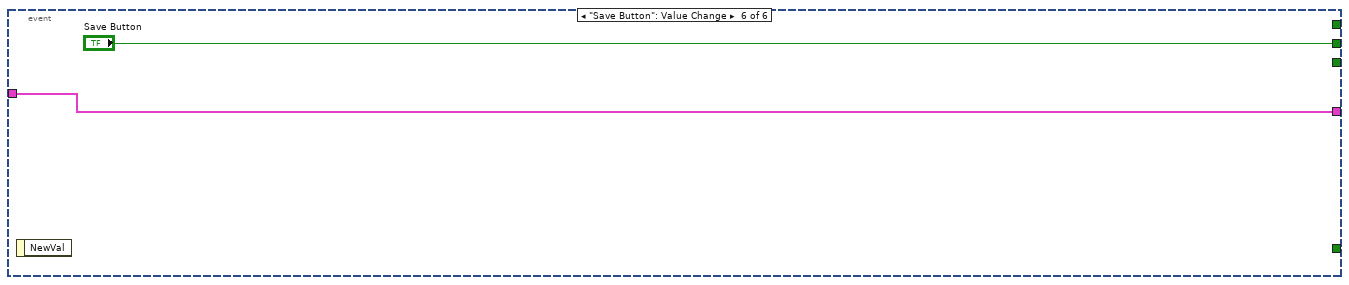
[diagram p16: hidden frame]
diagram:
  w6 = u32 14  # Max Number of Rows
  n1 = invoke on="State Cluster In" class="Clust (strict)" method="Reinit To Default"(error in="error in (no error)") -> (error out=w4:errorcluster)  [unwired: 2 in, 2 out]
  n2 = case shown="No Error" w4 {
    selector: w4 -> [w12 w256]
    tunnel: [w12 w256] -> w7
    tunnel: w6 -> [w11 _]
    tunnel: "State Cluster In" -> [w10 w255]
    tunnel: [w9 w255] -> w5
    tunnel: "Sequence UI" -> [w8 _]
    frame No Error {
      n3 = stacked-sequence {
        seq-local: [w63 _ _ _ _] -> [_ w141 _ _ _]
        seq-local: [w62 _ _ _ _] -> [_ w134 _ _ _]
        seq-local: [_ w141 _ _ _] -> [_ _ w161 _ _]
        seq-local: [_ w134 _ _ _] -> [_ _ w160 _ _]
        seq-local: [_ _ w161 _ _] -> [_ _ _ w164 _]
        seq-local: [_ _ w160 _ _] -> [_ _ _ w163 _]
        seq-local: [_ _ _ w163 _] -> [_ _ _ _ w233]
        seq-local: [_ _ _ w162 _] -> [_ _ _ _ w231]
        seq-local: [w13 _ _ _ _] -> [_ w128 _ _ w230]
        tunnel: w11 -> [w63 _ _ _ _]
        tunnel: w10 -> [w62 _ _ _ _]
        tunnel: [_ _ _ _ w234] -> w9
        tunnel: w8 -> [_ _ _ _ w229]
        frame #0 {
          w51 = refnum<vi> refnum  # Ring
          # "Populate the module dropdown"
          # "Find the names of all the modules that can be controlled from the Sequencer"
          # "0 = False\n1 = Latched Bool\n2 = Module\n3 = Control\n4 = Value\n5 = Wait"
          n4 = Unbundle By Name(w62) -> ("Main Config.Feed Module Configs"=w64:T19[], "Main Config.Pump Module Configs"=w41:T43[], "Main Config.TCU Module Configs"=w38:T49[], "Main Config.DO Module Configs"=w34:T56[], "Main Config.PR Module Configs"=w32:T61[], "Main Config.TT Module Configs"=w30:T36[], "Main Config.PT Module Configs"=w26:T40[], "Main Config.Scale Module Configs"=w21:T41[], "Main Config.Flow Module Configs"=w20:T47[])
          n5 = for {
            shift-right: [w124] -> w42
            shift-left: _ -> [w126]
            tunnel: w64 -> [w125] mode=indexing
            shift-right: [w123] -> w40
            shift-left: _ -> [w122]
            n6 = Unbundle By Name(w125) -> ("Process Name"=w127:string, "Queue Name"=w121:string)
            n7 = Build Array (concatenate)(w126, w127) -> (w124:string[])
            n8 = Build Array (concatenate)(w122, w121) -> (w123:string[])
          }
          n9 = for {
            shift-right: [w117] -> w37
            shift-left: w42 -> [w119]
            tunnel: w41 -> [w118] mode=indexing
            shift-right: [w116] -> w39
            shift-left: w40 -> [w115]
            n10 = Unbundle By Name(w118) -> ("Process Name"=w120:string, "Queue Name"=w114:string)
            n11 = Build Array (concatenate)(w119, w120) -> (w117:string[])
            n12 = Build Array (concatenate)(w115, w114) -> (w116:string[])
          }
          n13 = for {
            shift-right: [w110] -> w36
            shift-left: w37 -> [w112]
            tunnel: w38 -> [w111] mode=indexing
            shift-right: [w109] -> w35
            shift-left: w39 -> [w108]
            n14 = Unbundle By Name(w111) -> ("Process Name"=w113:string, "Queue Name"=w107:string)
            n15 = Build Array (concatenate)(w112, w113) -> (w110:string[])
            n16 = Build Array (concatenate)(w108, w107) -> (w109:string[])
          }
          n17 = control-ref of="Step Array"() -> (w57:refnum<vi>)
          n18 = property class="Arr"(reference=w57) -> ("Array Element"=w58:refnum<vi>)  [unwired: 1 in, 2 out]
          n19 = for {
            shift-right: [w104] -> w33
            shift-left: w36 -> [w105]
            shift-right: [w103] -> w31
            shift-left: w35 -> [w102]
            tunnel: w34 -> [w100] mode=indexing
            n20 = Unbundle By Name(w100) -> ("Process Name"=w106:string, "Queue Name"=w101:string)
            n21 = Build Array (concatenate)(w105, w106) -> (w104:string[])
            n22 = Build Array (concatenate)(w102, w101) -> (w103:string[])
          }
          n23 = for {
            shift-right: [w96] -> w28
            shift-left: w33 -> [w98]
            tunnel: w32 -> [w97] mode=indexing
            shift-right: [w95] -> w29
            shift-left: w31 -> [w94]
            n24 = Unbundle By Name(w97) -> ("Process Name"=w99:string, "Queue Name"=w93:string)
            n25 = Build Array (concatenate)(w98, w99) -> (w96:string[])
            n26 = Build Array (concatenate)(w94, w93) -> (w95:string[])
          }
          n27 = control-ref of="Add/Remove Cluster"() -> (w46:refnum<vi>)
          n28 = To More Specific Class(target class=w46, reference=w58) -> (specific class reference=w59:refnum<vi>)  [unwired: 1 in, 1 out]
          n29 = for {
            shift-right: [w89] -> w27
            shift-left: w28 -> [w91]
            tunnel: w30 -> [w90] mode=indexing
            shift-right: [w88] -> w25
            shift-left: w29 -> [w87]
            n30 = Unbundle By Name(w90) -> ("Process Name"=w92:string, "Queue Name"=w86:string)
            n31 = Build Array (concatenate)(w91, w92) -> (w89:string[])
            n32 = Build Array (concatenate)(w87, w86) -> (w88:string[])
          }
          n33 = property class="Clust"(reference=w59) -> ("Controls[]"=w52:refnum<vi>[])  [unwired: 1 in, 2 out]
          n34 = Index Array(array=w52, index #1=0 ("Index"), index #2=1 ("Index"), index #3=2 ("index"), index #4=3 ("index"), index #5=4 ("index"), index #6=5 ("index")) -> (element #3=w50:refnum<vi>)  [unwired: 5 out]
          n35 = for {
            shift-right: [w82] -> w23
            shift-left: w27 -> [w84]
            tunnel: w26 -> [w83] mode=indexing
            shift-right: [w81] -> w18
            shift-left: w25 -> [w80]
            n36 = Unbundle By Name(w83) -> ("Process Name"=w85:string, "Queue Name"=w79:string)
            n37 = Build Array (concatenate)(w84, w85) -> (w82:string[])
            n38 = Build Array (concatenate)(w80, w79) -> (w81:string[])
          }
          n39 = for {
            shift-right: [w75] -> w24
            shift-left: w23 -> [w77]
            tunnel: w21 -> [w76] mode=indexing
            shift-right: [w74] -> w22
            shift-left: w18 -> [w73]
            n40 = Unbundle By Name(w76) -> ("Process Name"=w78:string, "Queue Name"=w72:string)
            n41 = Build Array (concatenate)(w77, w78) -> (w75:string[])
            n42 = Build Array (concatenate)(w73, w72) -> (w74:string[])
          }
          n43 = for {
            shift-right: [w68] -> w19
            shift-left: w24 -> [w70]
            tunnel: w20 -> [w69] mode=indexing
            shift-right: [w67] -> w14
            shift-left: w22 -> [w66]
            n44 = Unbundle By Name(w69) -> ("Process Name"=w71:string, "Queue Name"=w65:string)
            n45 = Build Array (concatenate)(w70, w71) -> (w68:string[])
            n46 = Build Array (concatenate)(w66, w65) -> (w67:string[])
          }
          n47 = Build Array (concatenate)("Default", "Start Loop", "End Loop", w14) -> (w13:string[])
          n48 = Build Array (concatenate)("Default", "Start Loop", "End Loop", w19) -> (w47:string[])
          n49 = To More Specific Class(target class=w51, reference=w50) -> (specific class reference=w49:refnum<vi>, error out=w48:errorcluster)  [unwired: 1 in]
          n50 = property class="Ring"(reference=w49, error in=w48, "Strings []"=w47) -> ()  [unwired: 2 out]
        }
        frame #1 {
          # "If the Sequencer is not populated load it empty"
          # "If the Sequencer is already populated, load it"
          n51 = Unbundle By Name(w134) -> ("Main Config.Steps"=w135:T1)
          "Main Config.Steps" <- w135
          n52 = for {
            tunnel: w135 -> [w159] mode=indexing
            tunnel: [w158] -> w143 mode=indexing
            tunnel: w128 -> [w150]
            n53 = disable-structure shown="Enabled" {
              frame Disabled {
                n54 = property on="Module" class="Ring (strict)" props=["Strings []"]() -> ()  [unwired: 2 in, 3 out]
              }
              frame Enabled {
              }
            }
            n55 = Unbundle By Name(w159) -> ("Module"=w152:string, "Control"=w157:u16, "Value"=w156:dbl, "Wait (sec)"=w155:dbl)
            n56 = local read "Step Array"() -> (w154:T65[])
            n57 = Search 1D Array(1D array=w150, element=w152) -> (index of element=w151:i32)  [unwired: 1 in]
            n58 = Index Array(array=w154) -> (element=w153:T65)  [unwired: 1 in]
            n59 = Bundle By Name(cluster=w153, "Module"=w151, "Control"=w157, "Value"=w156, "Wait (sec)"=w155) -> (w158:T65)
            "Strings []" <- w150
          }
          n60 = Empty Array?(array=w143) -> (empty?=w144:bool)
          n61 = flat-sequence {
            tunnel: [w145] -> w132
            tunnel: w132 -> [w146]
            tunnel: [w146] -> w131
            tunnel: [w148] -> w133
            tunnel: w131 -> [w147]
            tunnel: [w147] -> w130
            tunnel: w130 -> [w149]
            frame #0 {
              n62 = local read "Step Array"() -> (w145:T65[])
            }
            frame #1 {
              n63 = invoke on="Step Array" class="Arr" method="Reinit To Default"() -> ()  [unwired: 3 in, 3 out]
            }
            frame #2 {
              n64 = local read "Step Array"() -> (w148:T65[])
            }
            frame #3 {
              n65 = local write "Step Array"(w149) -> ()
            }
          }
          n66 = Select(t=w133, s=w144, f=w143) -> (s? t:f=w129:T65[])
          n67 = Array Size(array=w129) -> (size(s)=w142:i32)
          n68 = Max & Min(x=w142, y=w141) -> (min(x,y)=w137:u32)  [unwired: 1 out]
          n69 = Greater?(x=w137, y=u32 1) -> (0:w139:bool)
          n70 = property on="Step Array" class="Arr"("Number of Rows"=w137, "HorizScroll"=FALSE ("Horizontal Scrollbar Visible"), "VertScroll"=w139, "Index Values"=u32[] [0], "Value"=w129) -> ()  [unwired: 2 in, 2 out]
        }
        frame #2 {
          n71 = invoke class="VI" method="FP.Open"() -> ()  [unwired: 5 in, 5 out]
        }
        frame #3 {
          n72 = while {
            tunnel: w164 -> [w172]
            shift-right: [w167] -> _
            shift-left: _ -> [w166]
            tunnel: [w165] -> w162
            stop <- w170 stop-if-true
            n73 = event shown="[0] \"Step Array\": Value Change" {
              selector: _ -> [_ _ _ _ _ _]
              dyn-events: _ -> [_ _ _ _ _ _]
              timeout: _ -> [_ _ _ _ _ _]
              tunnel: [_ "Start Button" "Cancel Button" "Abort  Button" TRUE ("Save Button") "Save Button"] -> w170
              tunnel: w172 -> [w176 _ _ _ _ _]
              tunnel: [_ _ "Cancel Button" _ _ _] -> w171
              tunnel: [_ "Start Button" _ _ _ _] -> w169
              tunnel: [_ _ _ _ "Pause Button" _] -> w168
              tunnel: [w174 w218 w220 w223 w224 w227] -> w167
              tunnel: w166 -> [_ w218 w220 w223 w224 w227]
              tunnel: [_ _ _ "Abort  Button" _ _] -> w165
              event "Step Array": Value Change {
                n74 = event-data() -> ("NewVal"=w173:T65[])  [unwired: 1 in]
                n75 = for {
                  tunnel: w173 -> [w212] mode=indexing
                  tunnel: [w213] -> w186 mode=indexing
                  tunnel: [w214] -> w185 mode=indexing
                  tunnel: [w211] -> w175 mode=indexing
                  workers-P: _ -> [_]
                  n76 = in-place {
                    in-place-border: [w216] -> w214
                    in-place-border: [w217] -> w213
                    w215 = FALSE ("Add Button")
                    n77 = in-place-cluster #1(w212) -> ("Add Button"=w217:bool, "Remove Button"=w216:bool)
                    n78 = in-place-cluster #1("Add Button"=w215, "Remove Button"=w215) -> (w211:T65)
                  }
                }
                n79 = Or Array Elements(Boolean array=w186) -> (logical OR=w187:bool)
                n80 = Or Array Elements(Boolean array=w185) -> (logical OR=w184:bool)
                n81 = case "Add?" shown="False" w187 {
                  tunnel: w186 -> [_ w210]
                  tunnel: w175 -> [w194 w208]
                  tunnel: [w193 w206] -> w174
                  tunnel: w185 -> [w196 _]
                  tunnel: w184 -> [w195 _]
                  tunnel: [_ w205] -> w177
                  frame False {
                    n82 = case "Remove?" shown="True" w195 {
                      tunnel: w196 -> [_ w202]
                      tunnel: w194 -> [w197 w201]
                      tunnel: [w197 w198] -> w193
                      frame False {
                      }
                      frame True {
                        n83 = Search 1D Array(1D array=w202, element=TRUE) -> (index of element=w199:i32)  [unwired: 1 in]
                        n84 = Delete From Array(array=w201, length=1, index=w199) -> (array with subset deleted=w198:T65[])  [unwired: 1 out]
                      }
                    }
                  }
                  frame True {
                    n85 = Search 1D Array(1D array=w210, element=TRUE) -> (index of element=w207:i32)  [unwired: 1 in]
                    n86 = Increment(x=w207) -> (x+1=w205:i32)
                    n87 = Insert Into Array(array=w208, index=w205, new element=T66 {"Add Button"=FALSE, "Remove Button"=FALSE, "Module"=0, "Control"=9, "Value"=0.0, "Wait (sec)"=0.0, "Step Running"=FALSE} ("Add/Remove Cluster")) -> (w206:T65[])
                  }
                }
                n88 = local write "Step Array"(w174) -> ()
                n89 = Greater Or Equal?(x=w177, y=w176) -> (x >= y?=w178:bool)
                n90 = Array Size(array=w174) -> (size(s)=w183:i32)
                n91 = case shown="True" w178 {
                  tunnel: w177 -> [_ w192]
                  tunnel: w176 -> [_ w191]
                  frame False {
                  }
                  frame True {
                    # "Keep last row in view"
                    n92 = Subtract(x=w192, y=w191) -> (x-y=w190:u32)
                    n93 = Increment(x=w190) -> (x+1=w189:u32)
                    n94 = Build Array(w189) -> (w188:u32[])
                    n95 = property on="Step Array" class="Arr"("Index Values"=w188) -> ()  [unwired: 2 in, 2 out]
                  }
                }
                n96 = Max & Min(x=w183, y=w176) -> (min(x,y)=w180:u32)  [unwired: 1 out]
                n97 = Greater?(x=w180, y=u32 1) -> (0:w179:bool)
                n98 = property on="Step Array" class="Arr"("Number of Rows"=w180, "HorizScroll"=FALSE ("Horizontal Scrollbar Visible"), "VertScroll"=w179) -> ()  [unwired: 2 in, 2 out]
              }
              event "Start Button": Value Change {
                n99 = event-data() -> ()  [unwired: 1 in, 1 out]
              }
              event "Cancel Button": Value Change {
                n100 = event-data() -> ()  [unwired: 1 in, 1 out]
              }
              event "Abort  Button": Value Change {
                n101 = event-data() -> ()  [unwired: 1 in, 1 out]
              }
              event "Pause Button": Value Change {
                n102 = event-data() -> ()  [unwired: 1 in, 1 out]
              }
              event "Save Button": Value Change {
                n103 = event-data() -> ()  [unwired: 1 in, 1 out]
              }
            }
            "cancelled" <- w171
            "Start" <- w169
            "Pause" <- w168
            "Abort" <- w165
          }
        }
        frame #4 {
          n104 = local read "cancelled"() -> (w235:bool)
          n105 = case shown="False" w235 {
            tunnel: w233 -> [w241 w254]
            tunnel: [w240 w254] -> w234
            tunnel: w233 -> [w239 _]
            tunnel: w231 -> [w238 _]
            tunnel: w230 -> [w237 _]
            frame False {
              # "Send out the Sequence"
              n106 = local read "Step Array"() -> (w242:T65[])
              n107 = for {
                tunnel: w242 -> [w253] mode=indexing
                tunnel: [w249] -> w236 mode=indexing
                tunnel: w239 -> [w244]
                tunnel: w237 -> [w243]
                n108 = Unbundle By Name(w244) -> ("Main Config.Steps"=w248:T1)
                n109 = Unbundle By Name(w253) -> ("Module"=w246:u16, "Control"=w252:u16, "Value"=w251:dbl, "Wait (sec)"=w250:dbl)
                n110 = property on="Module" class="Ring (strict)" props=["Strings []"]() -> ()  [unwired: 2 in, 3 out]
                n111 = Index Array(array=w248) -> (element=w247:T2)  [unwired: 1 in]
                n112 = Index Array(array=w243, index=w246) -> (element=w245:string)
                n113 = Bundle By Name(cluster=w247, "Module"=w245, "Control"=w252, "Value"=w251, "Wait (sec)"=w250) -> (w249:T2)
              }
              "Steps out" <- w236
              n114 = Bundle By Name(cluster=w241, "Main Config.Abort"=w238, "Main Config.Steps"=w236) -> (w240:T3)
            }
            frame True {
            }
          }
          n115 = invoke class="VI" method="FP.Close"() -> ()  [unwired: 3 in, 3 out]
          n116 = call-poly "Enqueue Message.vi"("Message"="Exit", "Message Queue"=w229) -> ()  [unwired: 8 in, 2 out]
        }
      }
    }
    frame Error {
    }
  }
  "error out" <- w7
  "State Cluster Out" <- w5
  n117 = while {
    tunnel: "Sequence UI" -> [w261]
    stop <- w260 stop-if-true
    n118 = call "Dequeue Message.vi"("Message Queue"=w261) -> ("Message Data"=w259:variant, "Message"=w262:string)  [unwired: 7 in, 2 out]
    n119 = Variant To Data(type=0, Variant=w259) -> (data=w257:i32)  [unwired: 1 in, 1 out]
    n120 = case shown="\"Exit\"" w262 {
      tunnel: [FALSE FALSE TRUE] -> w260
      tunnel: w257 -> [_ w266 _]
      frame Default {
        n121 = Wait (ms)(milliseconds to wait=u32 50) -> ()  [unwired: 1 out]
      }
      frame "Update Step" {
        n122 = local read "Step Array"() -> (w267:T65[])
        n123 = for {
          tunnel: w267 -> [w271] mode=indexing
          tunnel: w266 -> [w272]
          tunnel: [w270] -> w265 mode=indexing
          i -> [w273]
          n124 = Equal?(x=w273, y=w272) -> (x = y?=w269:bool)
          n125 = Bundle By Name(cluster=w271, "Step Running"=w269) -> (w270:T65)
        }
        n126 = local write "Step Array"(w265) -> ()
      }
      frame "Exit" {
      }
    }
  }
